vi "Get Excel Value.vi"(6 "SheetName(\"\")":string, 8 "error in (no error)":errorcluster, 9 "End":cluster{"Column":i32, "Row":i32}={"Column"=8, "Row"=7}, 10 "Start":cluster{"Column":i32, "Row":i32}={"Column"=1, "Row"=1}, 11 "path":path) -> (0 "error out":errorcluster, 2 "Excel_Value":variant)   [LabVIEW 2015]
uses:
  Private Methods/OpenXL_WorkSheet By Name.vi
  Private Methods/GetXL_CellValues_2D_String.vi
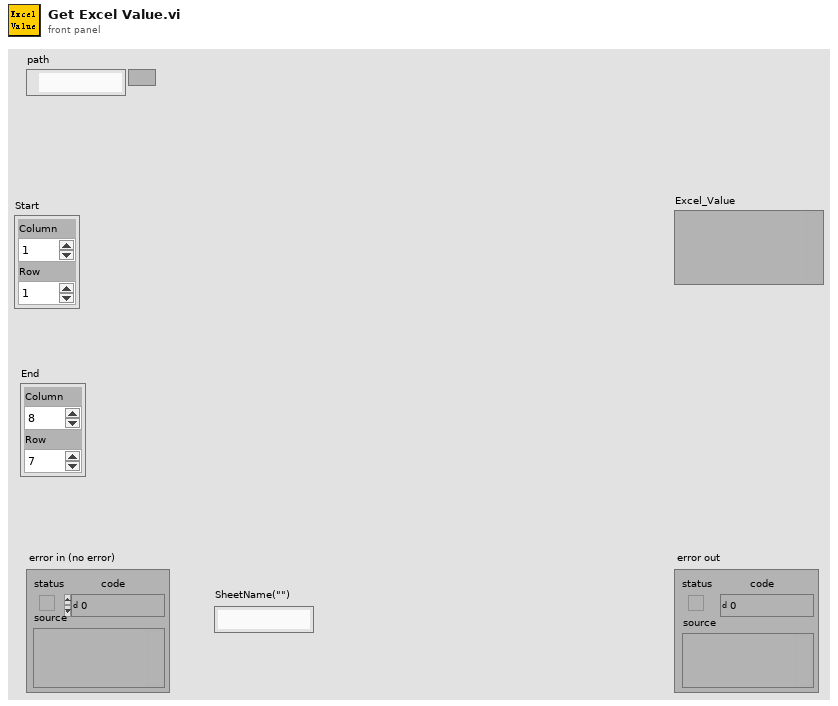
[diagram p1: front panel]
types:
  T1 = cluster{"Excel._Application":refnum<k7>, "Workbooks":refnum<k7>}
  T2 = cluster{"Excel._Application":refnum<k7>, "Workbooks":refnum<k7>, "Open":refnum<k7>}
  T3 = cluster{"Excel._Application":refnum<k7>, "Workbooks":refnum<k7>, "Open":refnum<k7>, "Worksheets":refnum<k7>, "Excel._Worksheet":refnum<k7>}
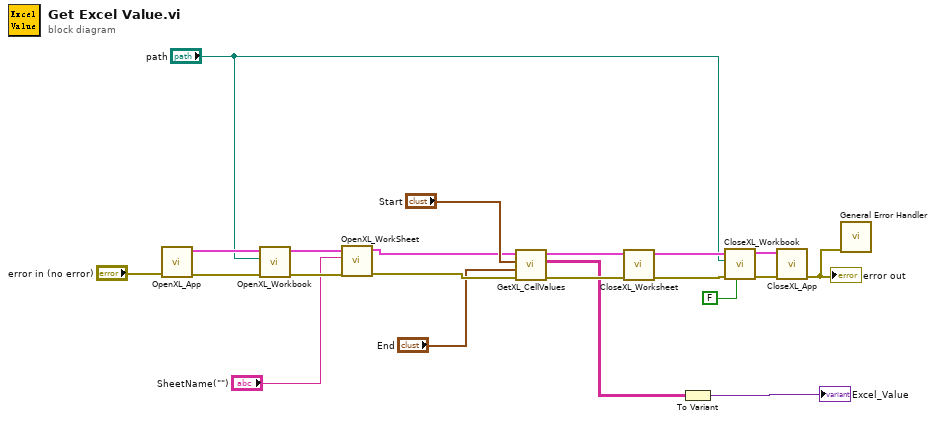
[diagram p0: block diagram]
diagram:
  n1 = call "OpenXL_App.vi"("error in (no error)"="error in (no error)") -> ("error out"=w20:errorcluster, "Refnum Cluster"=w21:T1)  [unwired: 9 in]
  n2 = call "OpenXL_Workbook.vi"("error in"=w20, "path"="path", "Refnum Cluster In"=w21) -> ("error out"=w10:errorcluster, "Refnum Cluster Out"=w11:T2)  [unwired: 7 in]
  n3 = call-poly "OpenXL_WorkSheet.vi"("error in (no error)"=w10, "SheetName(\"\")"="SheetName(\"\")", "Refnum Cluster In"=w11) -> ("error out"=w9:errorcluster, "Refnum Cluster Out"=w6:T3)  [unwired: 7 in]
  n4 = call-poly "GetXL_CellValues.vi"("error in"=w9, "End"="End", "Start"="Start", "Refnum Cluster In"=w6) -> ("error out"=w19:errorcluster, "data"=w5:string[][], "Refnum Cluster Out"=w18:T3)  [unwired: 5 in]
  n5 = call "CloseXL_Worksheet.vi"("error in (no error)"=w19, "Refnum Cluster In"=w18) -> ("error out"=w16:errorcluster, "Refnum Cluster Out"=w17:T2)  [unwired: 8 in]
  n6 = To Variant(anything=w5) -> (Variant=→"Excel_Value":variant)
  n7 = call "CloseXL_Workbook.vi"("Save? (F)"=FALSE, "error in (no error)"=w16, "path"="path", "Refnum Cluster In"=w17) -> ("error out"=w14:errorcluster, "Refnum Cluster Out"=w15:T1)  [unwired: 6 in]
  n8 = call "CloseXL_App.vi"("error in (no error)"=w14, "Refnum Cluster In"=w15) -> ("error out"=w1:errorcluster)  [unwired: 9 in]
  "error out" <- w1
  n9 = call <vilib>:"General Error Handler.vi"("error in (no error)"=w1) -> ()  [unwired: 10 in, 5 out]
